vi "LM 2D Gaussian + Blinking ACF and gradient.vi"(3 "output control":T1, 4 "data":variant, 5 "X":dbl[](array[numeric]), 6 "a":dbl[](array[numeric])) -> (0 "error out":errorcluster, 1 "f'(X,a)":dbl[][](array[numeric]), 2 "f(X,a)":dbl[](array[numeric]))   [LabVIEW 2021, in "Fits.lvlib"]
doc: "This template is the starting point for creating a model function to be passed to the Nonlinear Curve Fit.vi."
uses:
  <vilib>/gmath/NumericalOptimization/LM_output select.ctl
  Fits.lvlib
  <vilib>/gmath/NI_Gmath.lvlib
panel:
  # "Parameters:\n\namplitude: A\ndiffusion time: t1\nblinking fraction: b\nblinking time constant: t2"
  # "f(x) = 1 + A/(1+x/t1)*(1- b + b*Exp(-x/t2)"
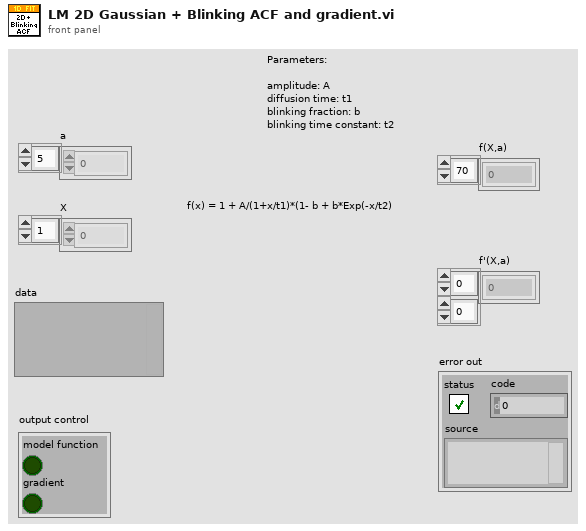
[diagram p1: front panel]
types:
  T1 = typedef "NI_Gmath.lvlib/LM_output select.ctl" = cluster{"model function":bool, "gradient":bool}
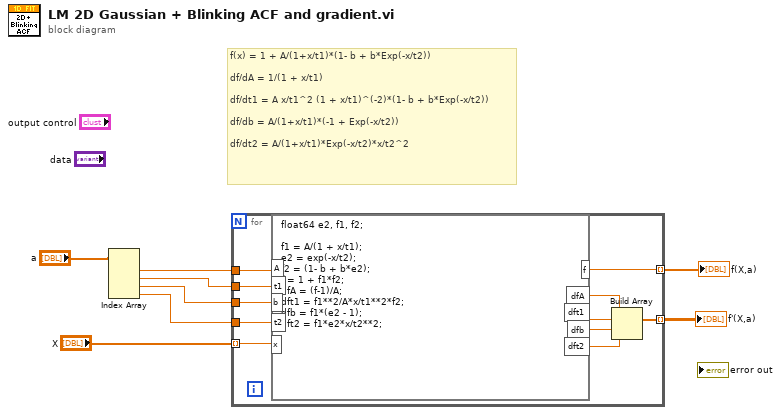
[diagram p0: block diagram]
diagram:
  # "f(x) = 1 + A/(1+x/t1)*(1- b + b*Exp(-x/t2))\n\ndf/dA = 1/(1 + x/t1)\n\ndf/dt1 = A x/t1^2 (1 + x/t1)^(-2)*(1- b + b*Exp(-x/t2))\n\ndf/db = A/(1+x/t1)*(-1 + Exp(-x/t2))\n\ndf/dt2 = A/(1+x/t1)*Exp(-x/t2)*x/t2^2"
  n1 = Index Array(array="a") -> (element #1=w4:dbl, element #2=w3:dbl, element #3=w2:dbl, element #4=w1:dbl)  [unwired: 4 in]
  n2 = for {
    tunnel: w4 -> [w18]
    tunnel: w3 -> [w19]
    tunnel: "X" -> [w17] mode=indexing
    tunnel: [w16] -> w6 mode=indexing
    tunnel: [w13] -> w5 mode=indexing
    tunnel: w2 -> [w12]
    tunnel: w1 -> [w11]
    n3 = formula code="float64 e2, f1, f2;\n\nf1 = A/(1 + x/t1);\ne2 = exp(-x/t2);\nf2 = (1- b + b*e2);\nf = 1 + f1*f2;\ndfA = (f-1)/A;\ndft1 = f1**2/A*x/t1**2*f2;\ndfb = f1*(e2 - 1);\ndft2 = f1*e2*x/t2**2;"("A"=w18, "t1"=w19, "x"=w17, "b"=w12, "t2"=w11) -> ("f"=w16:dbl, "dfA"=w15:dbl, "dft1"=w14:dbl, "dfb"=w10:dbl, "dft2"=w9:dbl)
    n4 = Build Array(w15, w14, w10, w9) -> (w13:dbl[])
  }
  "f(X,a)" <- w6
  "f'(X,a)" <- w5
